vi "AudioProtocol.vi"(0 "Array":string[](array[string])) -> (4 "modeAudio":string, 6 "xAudio":i32, 8 "yAudio":i32, 10 "xTV":i32, 15 "yTV":i32)   [LabVIEW 2018]
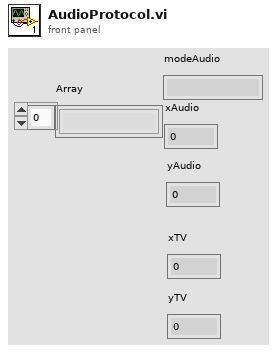
[diagram p1: front panel]
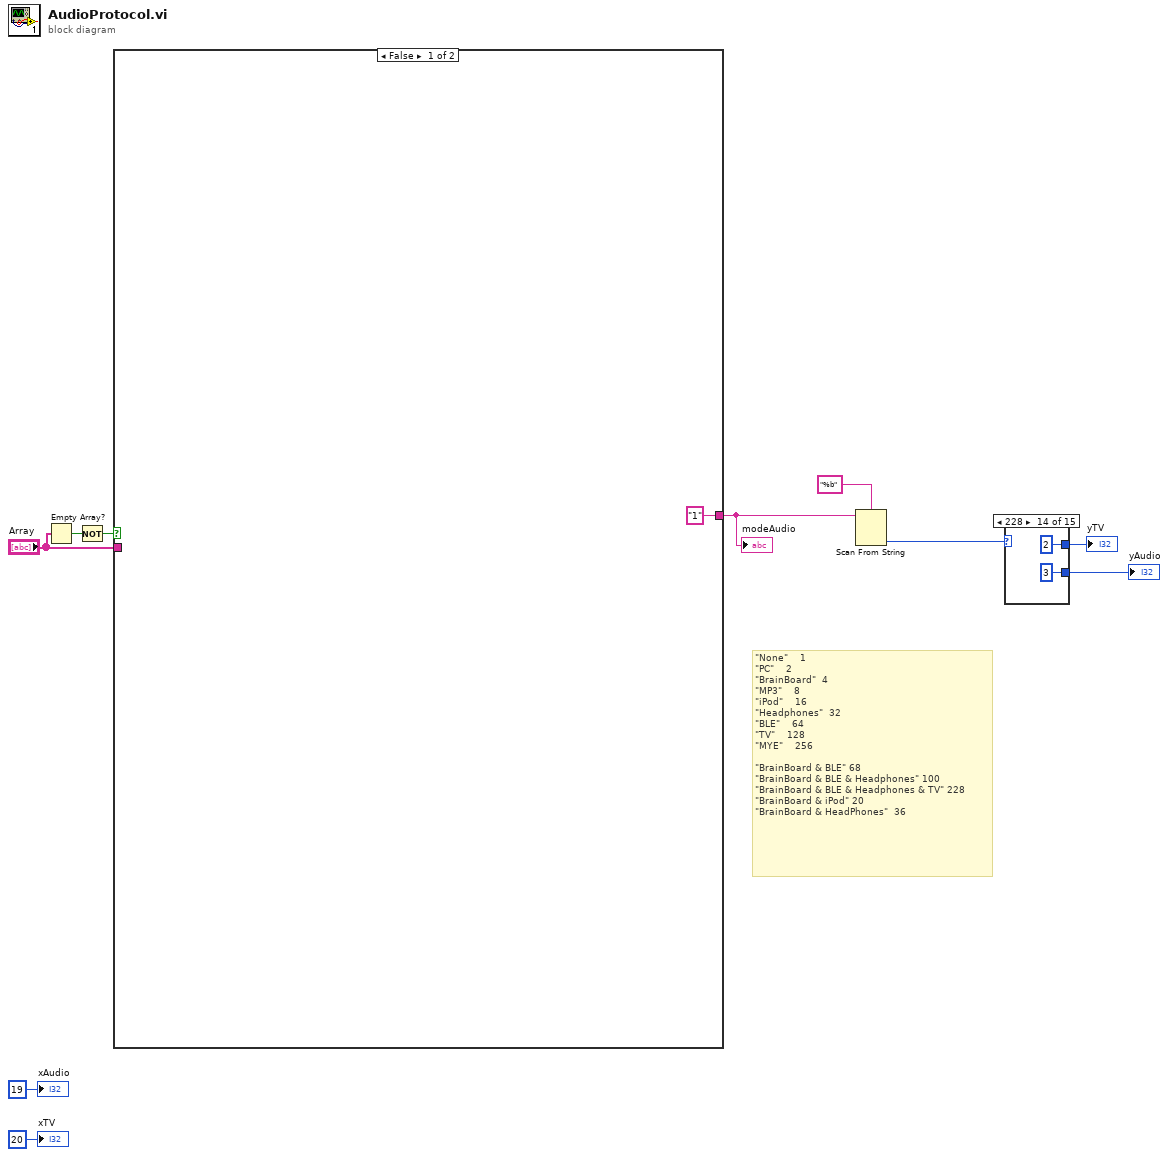
[diagram p0: block diagram]
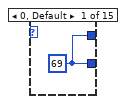
[diagram p2: hidden frame]
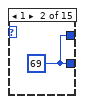
[diagram p3: hidden frame]
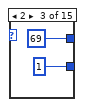
[diagram p4: hidden frame]
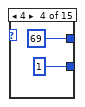
[diagram p5: hidden frame]
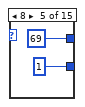
[diagram p6: hidden frame]
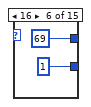
[diagram p7: hidden frame]
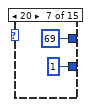
[diagram p8: hidden frame]
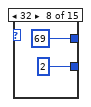
[diagram p9: hidden frame]
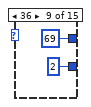
[diagram p10: hidden frame]
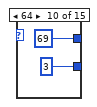
[diagram p11: hidden frame]
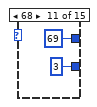
[diagram p12: hidden frame]
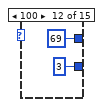
[diagram p13: hidden frame]
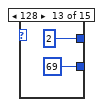
[diagram p14: hidden frame]
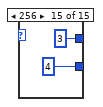
[diagram p15: hidden frame]
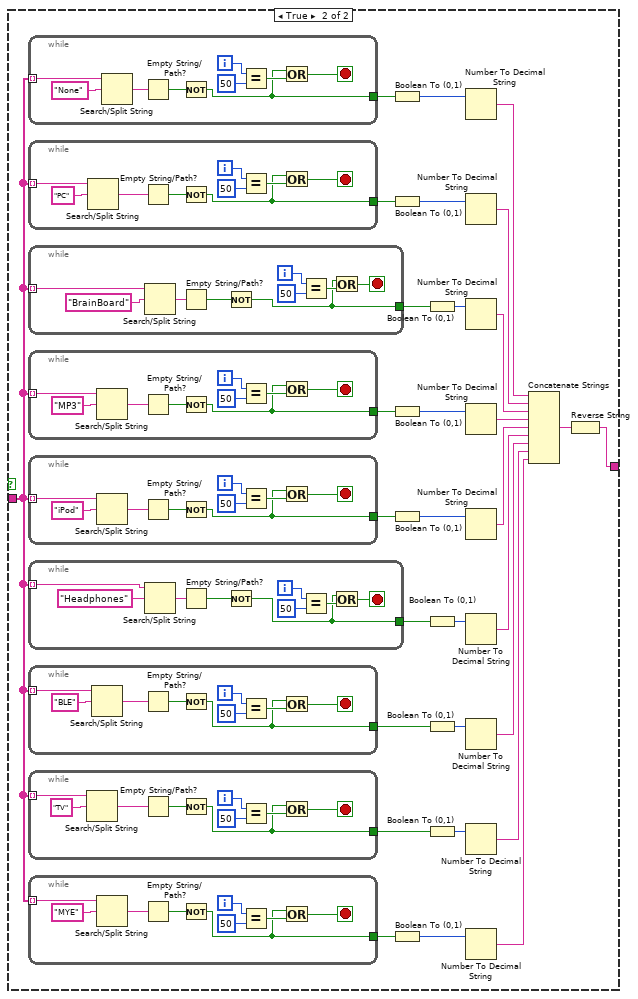
[diagram p16: hidden frame]
diagram:
  # "\"None\"\t\t\t\t1\n\"PC\"\t\t\t\t2\n\"BrainBoard\"\t\t4\n\"MP3\"\t\t\t\t8\n\"iPod\"\t\t\t\t16\n\"Headphones\"\t\t32\n\"BLE\"\t\t\t\t64\n\"TV\"\t\t\t\t128\n\"MYE\"\t\t\t\t256\n\n\"BrainBoard & BLE\"\t68\n\"BrainBoard & BLE & Headphones\"\t100\n\"BrainBoard & BLE & Headphones & TV\"\t228\n\"BrainBoard & iPod\" 20\n\"BrainBoard & HeadPhones\"  36"
  n1 = Empty Array?(array="Array") -> (empty?=w10:bool)
  n2 = Not(x=w10) -> (.not. x?=w9:bool)
  n3 = case shown="False" w9 {
    tunnel: "Array" -> [_ w17]
    tunnel: ["1" w12] -> w4
    frame False {
    }
    frame True {
      n4 = while {
        tunnel: w17 -> [w118] mode=indexing
        tunnel: [w114] -> w36
        i -> [w122]
        stop <- w120 stop-if-true
        n5 = Search/Split String(string=w118, search string/char (-)="None") -> (match + rest of string=w115:string)  [unwired: 1 in, 2 out]
        n6 = Empty String/Path?(string/path=w115) -> (empty?=w116:bool)
        n7 = Not(x=w116) -> (.not. x?=w114:bool)
        n8 = Equal?(x=w122, y=50) -> (x = y?=w119:bool)
        n9 = Or(x=w114, y=w119) -> (x .or. y?=w120:bool)
      }
      n10 = while {
        tunnel: w17 -> [w109] mode=indexing
        tunnel: [w105] -> w37
        i -> [w113]
        stop <- w111 stop-if-true
        n11 = Search/Split String(string=w109, search string/char (-)="PC") -> (match + rest of string=w106:string)  [unwired: 1 in, 2 out]
        n12 = Empty String/Path?(string/path=w106) -> (empty?=w107:bool)
        n13 = Not(x=w107) -> (.not. x?=w105:bool)
        n14 = Equal?(x=w113, y=50) -> (x = y?=w110:bool)
        n15 = Or(x=w105, y=w110) -> (x .or. y?=w111:bool)
      }
      n16 = while {
        tunnel: w17 -> [w100] mode=indexing
        tunnel: [w96] -> w38
        i -> [w104]
        stop <- w102 stop-if-true
        n17 = Search/Split String(string=w100, search string/char (-)="BrainBoard") -> (match + rest of string=w97:string)  [unwired: 1 in, 2 out]
        n18 = Empty String/Path?(string/path=w97) -> (empty?=w98:bool)
        n19 = Not(x=w98) -> (.not. x?=w96:bool)
        n20 = Equal?(x=w104, y=50) -> (x = y?=w101:bool)
        n21 = Or(x=w96, y=w101) -> (x .or. y?=w102:bool)
      }
      n22 = while {
        tunnel: w17 -> [w91] mode=indexing
        tunnel: [w87] -> w30
        i -> [w95]
        stop <- w93 stop-if-true
        n23 = Search/Split String(string=w91, search string/char (-)="MP3") -> (match + rest of string=w88:string)  [unwired: 1 in, 2 out]
        n24 = Empty String/Path?(string/path=w88) -> (empty?=w89:bool)
        n25 = Not(x=w89) -> (.not. x?=w87:bool)
        n26 = Equal?(x=w95, y=50) -> (x = y?=w92:bool)
        n27 = Or(x=w87, y=w92) -> (x .or. y?=w93:bool)
      }
      n28 = while {
        tunnel: w17 -> [w82] mode=indexing
        tunnel: [w78] -> w29
        i -> [w86]
        stop <- w84 stop-if-true
        n29 = Search/Split String(string=w82, search string/char (-)="iPod") -> (match + rest of string=w79:string)  [unwired: 1 in, 2 out]
        n30 = Empty String/Path?(string/path=w79) -> (empty?=w80:bool)
        n31 = Not(x=w80) -> (.not. x?=w78:bool)
        n32 = Equal?(x=w86, y=50) -> (x = y?=w83:bool)
        n33 = Or(x=w78, y=w83) -> (x .or. y?=w84:bool)
      }
      n34 = while {
        tunnel: w17 -> [w73] mode=indexing
        tunnel: [w69] -> w28
        i -> [w77]
        stop <- w75 stop-if-true
        n35 = Search/Split String(string=w73, search string/char (-)="Headphones") -> (match + rest of string=w70:string)  [unwired: 1 in, 2 out]
        n36 = Empty String/Path?(string/path=w70) -> (empty?=w71:bool)
        n37 = Not(x=w71) -> (.not. x?=w69:bool)
        n38 = Equal?(x=w77, y=50) -> (x = y?=w74:bool)
        n39 = Or(x=w69, y=w74) -> (x .or. y?=w75:bool)
      }
      n40 = while {
        tunnel: w17 -> [w64] mode=indexing
        tunnel: [w60] -> w27
        i -> [w68]
        stop <- w66 stop-if-true
        n41 = Search/Split String(string=w64, search string/char (-)="BLE") -> (match + rest of string=w61:string)  [unwired: 1 in, 2 out]
        n42 = Empty String/Path?(string/path=w61) -> (empty?=w62:bool)
        n43 = Not(x=w62) -> (.not. x?=w60:bool)
        n44 = Equal?(x=w68, y=50) -> (x = y?=w65:bool)
        n45 = Or(x=w60, y=w65) -> (x .or. y?=w66:bool)
      }
      n46 = while {
        tunnel: w17 -> [w55] mode=indexing
        tunnel: [w51] -> w26
        i -> [w59]
        stop <- w57 stop-if-true
        n47 = Search/Split String(string=w55, search string/char (-)="TV") -> (match + rest of string=w52:string)  [unwired: 1 in, 2 out]
        n48 = Empty String/Path?(string/path=w52) -> (empty?=w53:bool)
        n49 = Not(x=w53) -> (.not. x?=w51:bool)
        n50 = Equal?(x=w59, y=50) -> (x = y?=w56:bool)
        n51 = Or(x=w51, y=w56) -> (x .or. y?=w57:bool)
      }
      n52 = while {
        tunnel: w17 -> [w46] mode=indexing
        tunnel: [w42] -> w15
        i -> [w50]
        stop <- w48 stop-if-true
        n53 = Search/Split String(string=w46, search string/char (-)="MYE") -> (match + rest of string=w43:string)  [unwired: 1 in, 2 out]
        n54 = Empty String/Path?(string/path=w43) -> (empty?=w44:bool)
        n55 = Not(x=w44) -> (.not. x?=w42:bool)
        n56 = Equal?(x=w50, y=50) -> (x = y?=w47:bool)
        n57 = Or(x=w42, y=w47) -> (x .or. y?=w48:bool)
      }
      n58 = Boolean To (0,1)(Boolean=w36) -> (0, 1=w39:i16)
      n59 = Boolean To (0,1)(Boolean=w37) -> (0, 1=w40:i16)
      n60 = Boolean To (0,1)(Boolean=w30) -> (0, 1=w35:i16)
      n61 = Boolean To (0,1)(Boolean=w29) -> (0, 1=w34:i16)
      n62 = Boolean To (0,1)(Boolean=w15) -> (0, 1=w16:i16)
      n63 = Boolean To (0,1)(Boolean=w38) -> (0, 1=w41:i16)
      n64 = Boolean To (0,1)(Boolean=w28) -> (0, 1=w33:i16)
      n65 = Boolean To (0,1)(Boolean=w27) -> (0, 1=w32:i16)
      n66 = Boolean To (0,1)(Boolean=w26) -> (0, 1=w31:i16)
      n67 = Number To Decimal String(number=w39) -> (decimal integer string=w18:string)  [unwired: 1 in]
      n68 = Number To Decimal String(number=w40) -> (decimal integer string=w19:string)  [unwired: 1 in]
      n69 = Number To Decimal String(number=w41) -> (decimal integer string=w20:string)  [unwired: 1 in]
      n70 = Number To Decimal String(number=w35) -> (decimal integer string=w21:string)  [unwired: 1 in]
      n71 = Number To Decimal String(number=w34) -> (decimal integer string=w22:string)  [unwired: 1 in]
      n72 = Number To Decimal String(number=w33) -> (decimal integer string=w23:string)  [unwired: 1 in]
      n73 = Number To Decimal String(number=w32) -> (decimal integer string=w24:string)  [unwired: 1 in]
      n74 = Number To Decimal String(number=w31) -> (decimal integer string=w25:string)  [unwired: 1 in]
      n75 = Number To Decimal String(number=w16) -> (decimal integer string=w14:string)  [unwired: 1 in]
      n76 = Concatenate Strings(w18, w19, w20, w21, w22, w23, w24, w25, w14) -> (w13:string)
      n77 = Reverse String(1:w13) -> (0:w12:string)
    }
  }
  "modeAudio" <- w4
  n78 = Scan From String(format string="%b", input string=w4) -> (output 1=w5:i32)  [unwired: 3 in, 3 out]
  n79 = case shown="228" w5 {
    tunnel: [w123 w124 1 1 1 1 1 2 2 3 3 3 69 3 4] -> w6
    tunnel: [w123 w124 69 69 69 69 69 69 69 69 69 69 2 2 3] -> w3
    frame 0, Default {
      w123 = 69
    }
    frame 1 {
      w124 = 69
    }
    frame 2 {
    }
    frame 4 {
    }
    frame 8 {
    }
    frame 16 {
    }
    frame 20 {
    }
    frame 32 {
    }
    frame 36 {
    }
    frame 64 {
    }
    frame 68 {
    }
    frame 100 {
    }
    frame 128 {
    }
    frame 228 {
    }
    frame 256 {
    }
  }
  "yAudio" <- w6
  "yTV" <- w3
  "xAudio" <- 19 ("xAudio")
  "xTV" <- 20 ("xTV")
